vi "230427_Database_read_write.vi"() -> ()   [LabVIEW 2022 SP3]
uses:
  <vilib>/addons/database/Connection.llb/DB Tools Open Connec (Path).vi
  <vilib>/Utility/error.llb/Error Cluster From Error Code.vi
  <vilib>/addons/database/_DB Variant To Data/Database Variant To Data.xnode
  <vilib>/ErrorRing/Error Ring.xnode
  <vilib>/addons/database/NI_Database_API.lvlib
panel:
  in  "lnr":i32
  in  "strasse_nr":string
  in  "plz":string
  out "error out":errorcluster
  in  "error in (no error)":errorcluster
  in  "Write":bool
  in  "tel_nr":string
  in  "vertreter":string
  in  "strasse":string
  in  "ort":string
  in  "firma":string
  in  "stop":bool
  in  "Read":bool
  out "data":string[][](array[string])
  in  "table":string="lieferant"
  in  "connection information":path=path "D:/School/AIIT/4AHME/LabView/230427_Database_Access/230427_article_supplier.udl"
  # "Neuer Datensatz"
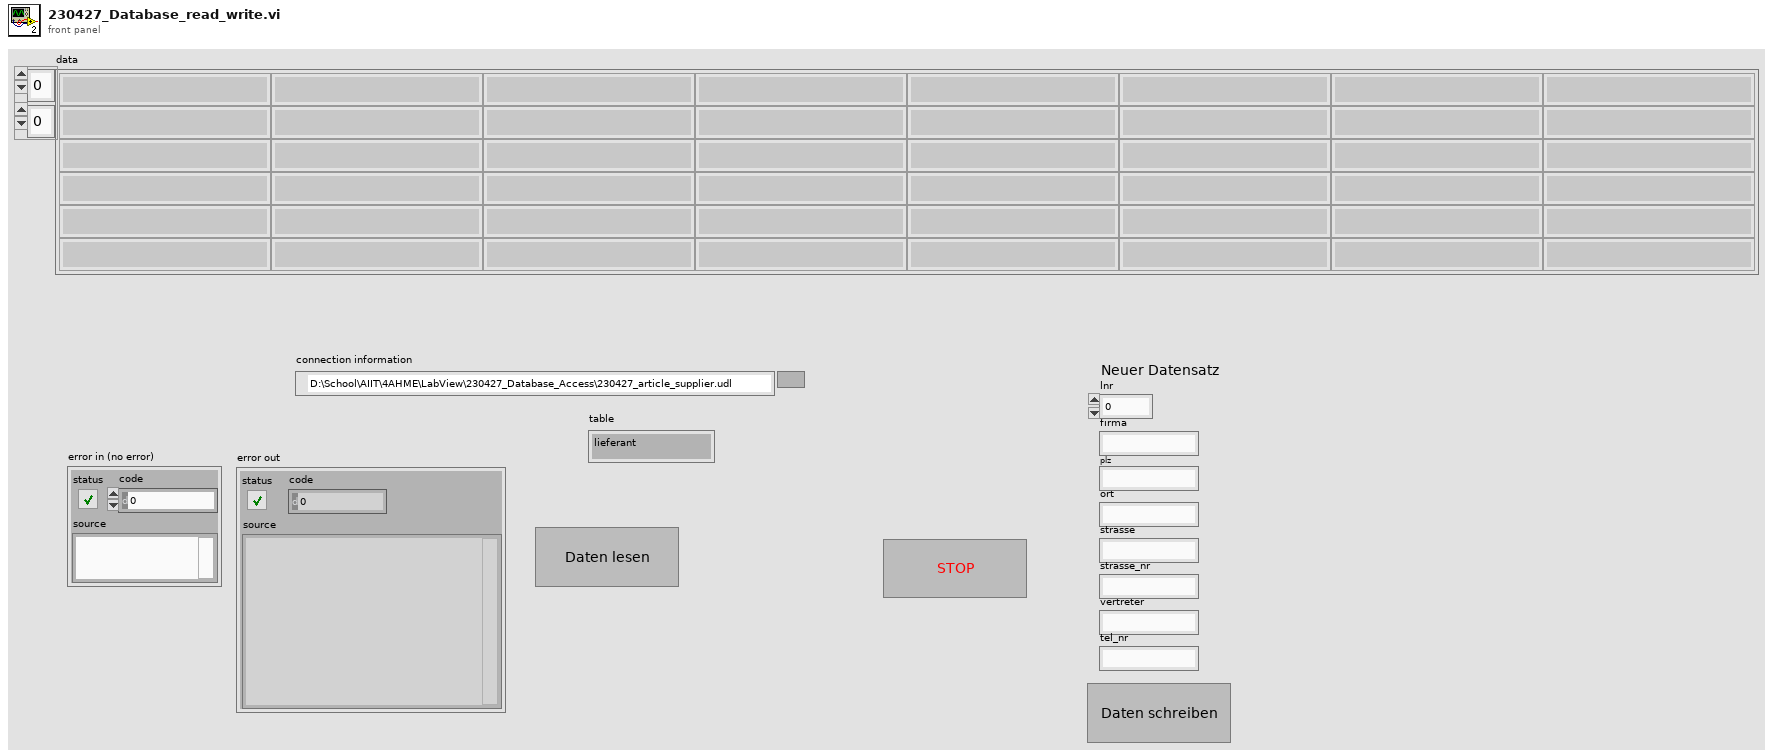
[diagram p1: front panel]
types:
  T1 = cluster{"firmenname":string, "plz":string, "ort":string, "strasse":string, "strasse_nr":string, "vertreter":string, "vertreter_tel_nr":string, "lnr":i32}
  T2 = typedef "NI_Database_API.lvlib/Conn ObjectReference.ctl" = refnum<k1>
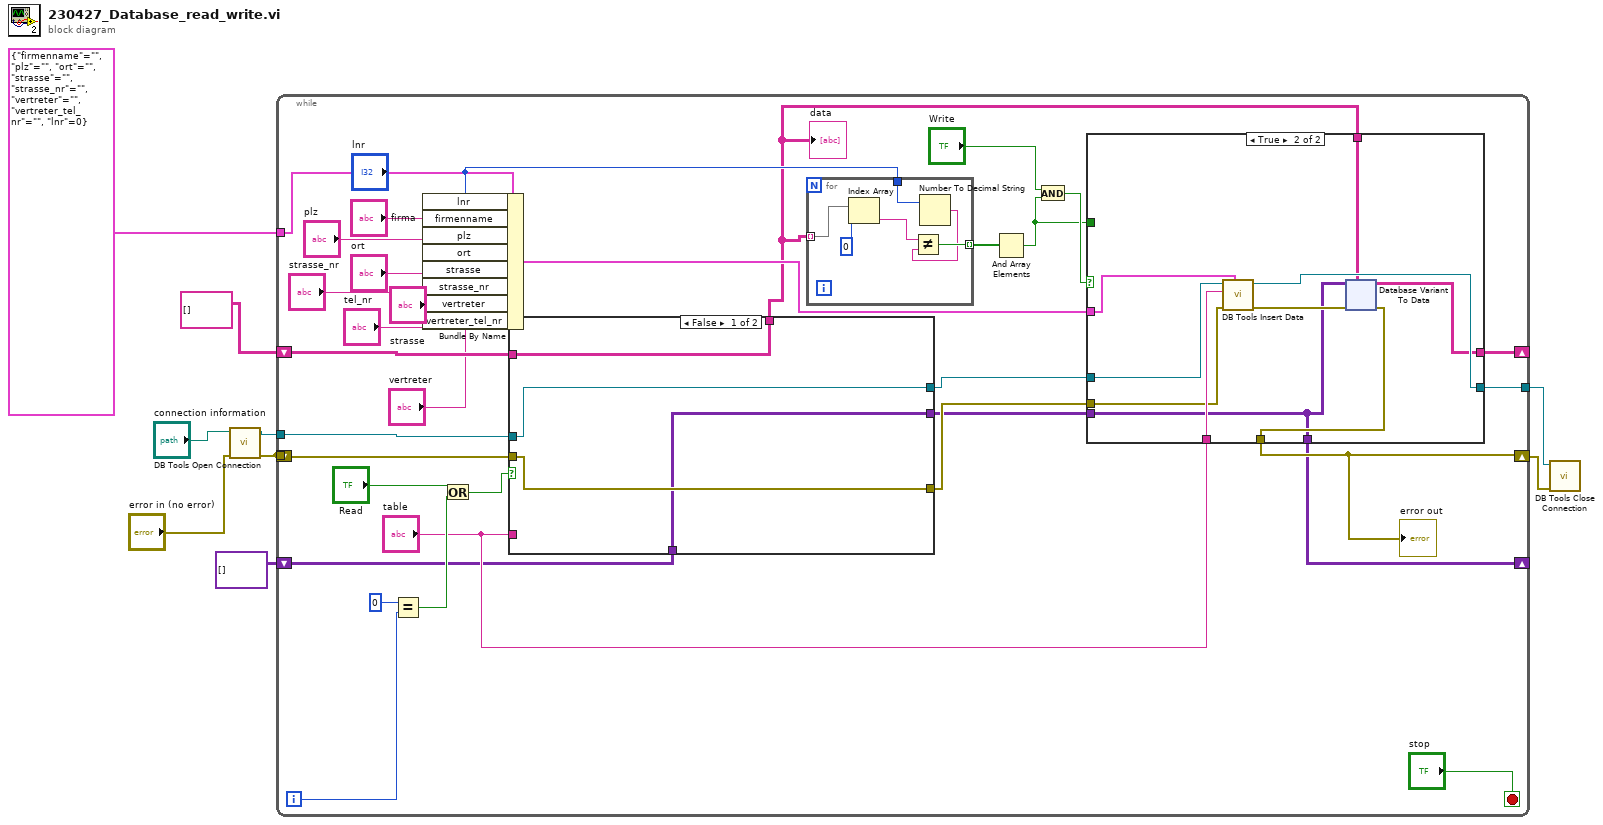
[diagram p0: block diagram]
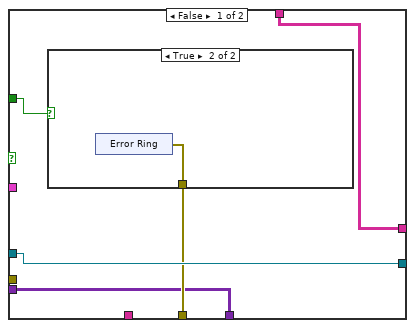
[diagram p2: hidden frame]
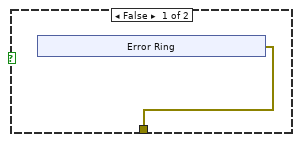
[diagram p3: hidden frame]
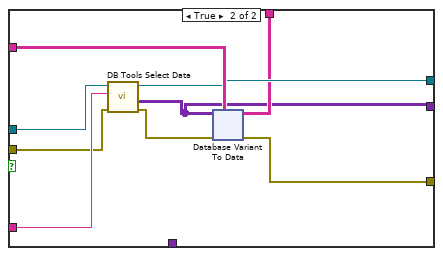
[diagram p4: hidden frame]
diagram:
  n1 = call-poly <vilib>:"DB Tools Open Connection.vi"("error in (no error)"="error in (no error)", "connection information"="connection information") -> ("error out"=w4:errorcluster, "connection reference"=w8:T2)  [unwired: 6 in]
  n2 = while {
    tunnel: w8 -> [w42]
    tunnel: w4 -> [_]
    tunnel: [w23] -> w6
    tunnel: T1 {"firmenname"="", "plz"="", "ort"="", "strasse"="", "strasse_nr"="", "vertreter"="", "vertreter_tel_nr"="", "lnr"=0} -> [w34]
    shift-right: [w17] -> w3
    shift-left: w4 -> [w19]
    shift-right: [w14] -> _
    shift-left: string[][] [] -> [w41]
    shift-right: [w13] -> _
    shift-left: variant[][] [] ("data") -> [w12]
    i -> [w39]
    stop <- "stop" stop-if-true
    n3 = Equal?(x=0, y=w39) -> (x = y?=w37:bool)
    n4 = Bundle By Name(cluster=w34, "lnr"="lnr", "firmenname"="firma", "plz"="plz", "ort"="ort", "strasse"="strasse", "strasse_nr"="strasse_nr", "vertreter"="vertreter", "vertreter_tel_nr"="tel_nr") -> (w22:T1)
    n5 = Or(x="Read", y=w37) -> (x .or. y?=w40:bool)
    n6 = case shown="False" w40 {
      tunnel: w42 -> [w119 w128]
      tunnel: w41 -> [w117 w127]
      tunnel: [w118 w125] -> w20
      tunnel: [w119 w124] -> w24
      tunnel: [w117 w123] -> w15
      tunnel: "table" -> [_ w122]
      tunnel: w19 -> [w118 w121]
      tunnel: [w116 w120] -> w16
      tunnel: w12 -> [w116 _]
      frame False {
      }
      frame True {
        n7 = call <vilib>:"DB Tools Select Data.vi"("error in (no error)"=w121, "table"=w122, "connection reference"=w128) -> ("error out"=w126:errorcluster, "data"=w120:variant[][], "connection reference out"=w124:T2)  [unwired: 3 in]
        n8 = xnode "Database Variant To Data"("database variant"=w120, "error in (no error)"=w126, "type"=w127) -> ("data"=w123:string[][], "error out"=w125:errorcluster)
      }
    }
    "data" <- w15
    n9 = for {
      tunnel: w15 -> [w115] mode=indexing
      tunnel: "lnr" -> [w111]
      tunnel: [w112] -> w27 mode=indexing
      n10 = Index Array(array=w115, index=0) -> (element=w113:string)
      n11 = Number To Decimal String(number=w111) -> (decimal integer string=w110:string)  [unwired: 1 in]
      n12 = Not Equal?(x=w113, y=w110) -> (x != y?=w112:bool)
    }
    n13 = And Array Elements(Boolean array=w27) -> (logical AND=w18:bool)
    n14 = And(x="Write", y=w18) -> (x .and. y?=w25:bool)
    n15 = case shown="True" w25 {
      tunnel: w24 -> [w47 w65]
      tunnel: [w47 w59] -> w23
      tunnel: w22 -> [_ w63]
      tunnel: "table" -> [_ w64]
      tunnel: w20 -> [_ w62]
      tunnel: [w46 w60] -> w17
      tunnel: w18 -> [w45 _]
      tunnel: w16 -> [w43 w56]
      tunnel: w15 -> [w44 w58]
      tunnel: [w44 w57] -> w14
      tunnel: [w43 w56] -> w13
      frame False {
        n16 = case shown="True" w45 {
          tunnel: [w48 w54] -> w46
          frame False {
            n17 = xnode "Error Ring"() -> ("error out"=w48:errorcluster)
          }
          frame True {
            n18 = xnode "Error Ring"() -> ("error out"=w54:errorcluster)
          }
        }
      }
      frame True {
        n19 = call <vilib>:"DB Tools Insert Data.vi"("data"=w63, "error in (no error)"=w62, "table"=w64, "connection reference"=w65) -> ("error out"=w61:errorcluster, "connection reference out"=w59:T2)  [unwired: 6 in]
        n20 = xnode "Database Variant To Data"("database variant"=w56, "error in (no error)"=w61, "type"=w58) -> ("data"=w57:string[][], "error out"=w60:errorcluster)
      }
    }
    "error out" <- w17
  }
  n21 = call <vilib>:"DB Tools Close Connection.vi"("error in (no error)"=w3, "connection reference"=w6) -> ()  [unwired: 5 in, 1 out]
